vi "DeferPanelUpdate.vi"(8 "error in (no error)":errorcluster, 10 "Defer Panel Updates (T)":bool=TRUE, 11 "Control in":refnum<vi>) -> (0 "error out":errorcluster, 2 "Defer Panel Updates Old":bool, 3 "Control out":refnum<vi>)   [LabVIEW 2021]
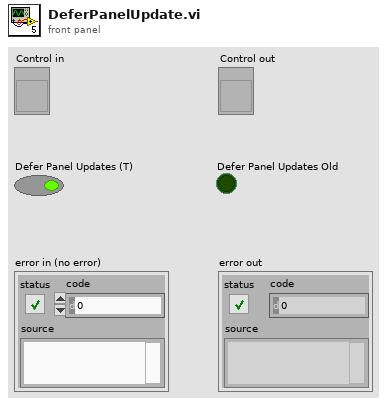
[diagram p1: front panel]
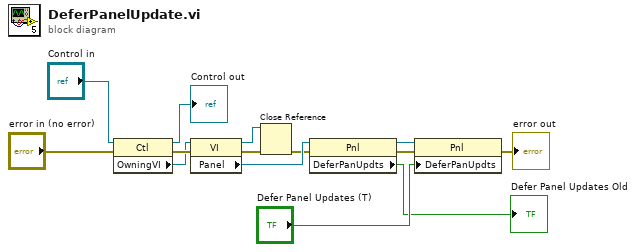
[diagram p0: block diagram]
diagram:
  n1 = property class="Ctl"(reference="Control in", error in="error in (no error)") -> (reference out=→"Control out":refnum<vi>, error out=w11:errorcluster, "OwningVI"=w10:refnum<vi>)
  n2 = property class="VI"(reference=w10, error in=w11) -> (reference out=w3:refnum<vi>, error out=w2:errorcluster, "Panel"=w7:refnum<vi>)
  n3 = Close Reference(reference=w3, error in (no error)=w2) -> (error out=w1:errorcluster)
  n4 = property class="Pnl"(reference=w7, error in=w1) -> (reference out=w5:refnum<vi>, error out=w6:errorcluster, "DeferPanUpdts"=→"Defer Panel Updates Old":bool)
  n5 = property class="Pnl"(reference=w5, error in=w6, "DeferPanUpdts"="Defer Panel Updates (T)") -> (error out=→"error out":errorcluster)  [unwired: 1 out]
